vi "niRFUtil MASMT Util Unconstained Linear Fit (DBL).vi"(0 "Y":dbl[](array[numeric]) format="%#.6g", 1 "method":i32(ring) items=["Least Square", "Least Absolute Residual", "Bisquare"], 5 "X":dbl[](array[numeric]) format="%#.6g", 7 "Weight":dbl[](array[numeric]) format="%#.6g", 9 "tolerance":dbl=9.999999747378752e-05, 11 "error in (no error)":errorcluster) -> (4 "Best Linear Fit":dbl[](array[numeric]) format="%#.6g", 6 "slope":dbl format="%#.6g", 8 "intercept":dbl format="%#.6g", 10 "residue":dbl format="%#.6g", 15 "error out":errorcluster)   [LabVIEW 2015, in "niRFUtil.lvlib"]
uses:
  niRFUtil.lvlib
  niRFMASMT_LINALG.dll
panel:
  out "Work":dbl[](array[numeric])
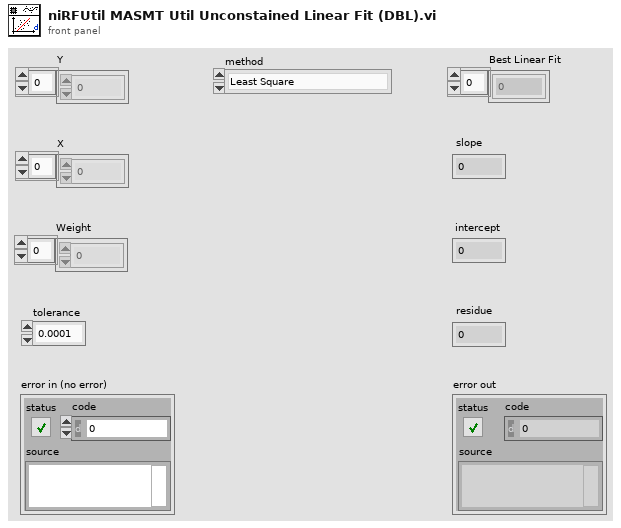
[diagram p1: front panel]
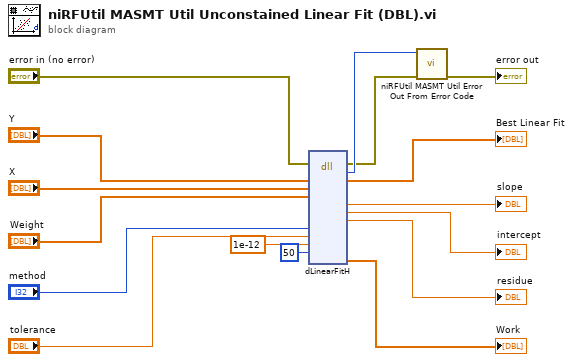
[diagram p0: block diagram]
diagram:
  n1 = dll-call lib="C:/Perforce/semoore-sales/Customers/NATI-3813/Noise Floor/LV Filters/ParallelComplexFilterRFUtil/niRFUtil/MASMT/Utilities/niRFMASMT_LINALG.*" fn="dLinearFitH"(error in="error in (no error)", "yH"="Y", "xH"="X", "weightH"="Weight", "method"="method", "relTol"="tolerance", "absTol"=1e-12, "maxIter"=50) -> (error out=w10:errorcluster, "return type"=w11:i32, "yH"=→"Best Linear Fit":dbl[], "slope"=→"slope":dbl, "intercept"=→"intercept":dbl, "residue"=→"residue":dbl, "WorkH"=→"Work":dbl[])  [unwired: 12 in, 1 out]
  n2 = call "niRFUtil MASMT Util Error Out From Error Code.vi"("error in (no error)"=w10, "error code"=w11) -> ("error out"=→"error out":errorcluster)  [unwired: 9 in]
